vi "TestLibLoadChecksumFile.vi"() -> ()   [LabVIEW 2020]
uses:
  TestLabviewTools32.dll
panel:
  out "RecordCount":u32
  out "ErrorOut":errorcluster
  out "FilePathOut":string
  out "Array":T1(array[cluster]) {"Checksum" format="%04x"}
  out "Result":i32
  in  "FilePath":path=path "C:/Factory/FactoryProductTestTool/FPTT_Checksum.lst"
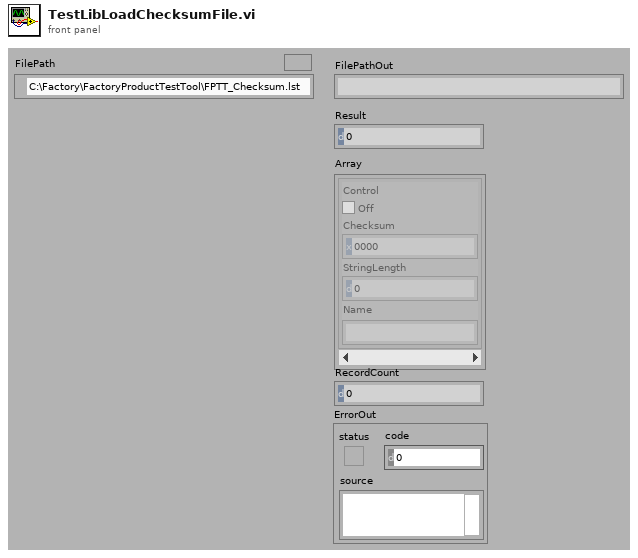
[diagram p1: front panel]
types:
  T1 = cluster{"Control":bool, "Checksum":u16, "StringLength":u32, "Name":string}[]
  T2 = cluster{bool, "Checksum":u16, "StringLength":u32, "Name":string}[]
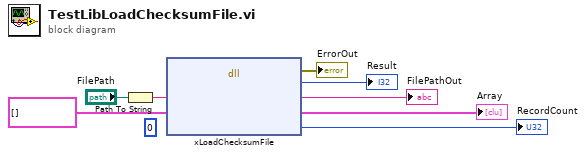
[diagram p0: block diagram]
diagram:
  (unwired) u32 0 ("vRecordCount")
  n1 = Path To String(path="FilePath") -> (string=w7:string)
  n2 = dll-call lib="C:/Factory/FactoryGenericTools/Dll/TestLabviewTools32.dll" fn="xLoadChecksumFile"("cFilePath"=w7, "vDataArray"=T2 [] ("Array")) -> (error out=→"ErrorOut":errorcluster, "fResult"=→"Result":i32, "cFilePath"=→"FilePathOut":string, "vDataArray"=→"Array":T2, "vRecordCount"=→"RecordCount":u32)  [unwired: 4 in, 1 out]
